vi "DevicePXIStar.vi"(11 "Channel Name":string) -> (2 "Trigger Source":string, 3 "PXIStarLine":string)   [LabVIEW 2014]
doc: "Takes a DAQmx Channel Name identifies the DAQmx device and outputs the device's PXI_Star port line and the PXI_Star line the device is connected to in the chasis.\n\nPXI_Star line of the device is the /\"device_name\"/PXI_Star \nPXI_Star line number is the slot number of the device minus 3."
uses:
  <resource>/objmgr/daqmx.rc
panel:
  out "PXI/PCI Settings:Slot Path":string
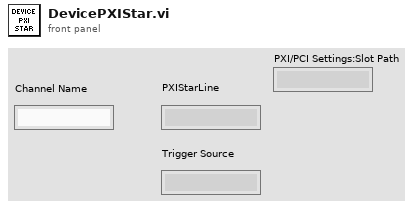
[diagram p1: front panel]
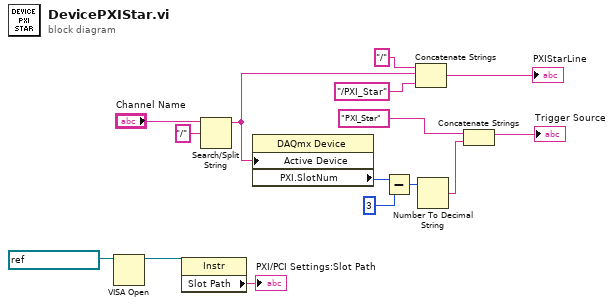
[diagram p0: block diagram]
diagram:
  n1 = VISA Open(VISA resource name=refnum<visa-resource-name> "RIO0::INSTR") -> (VISA resource name=w3:refnum<visa-resource-name>)  [unwired: 4 in, 1 out]
  n2 = property class="Instr"(reference=w3) -> ("Slot Path"=→"PXI/PCI Settings:Slot Path":string)  [unwired: 1 in, 2 out]
  n3 = Search/Split String(string="Channel Name", search string/char (-)="/") -> (substring before match=w6:string)  [unwired: 1 in, 2 out]
  n4 = property class="DAQmx Device"("Active Device"=w6) -> ("PXI.SlotNum"=w10:u32)  [unwired: 2 in, 2 out]
  n5 = Subtract(x=w10, y=u32 3) -> (x-y=w12:u32)
  n6 = Concatenate Strings("/" ("string"), w6, "/PXI_Star" ("string")) -> (→"PXIStarLine":string)
  n7 = Number To Decimal String(number=w12) -> (decimal integer string=w13:string)  [unwired: 1 in]
  n8 = Concatenate Strings("PXI_Star" ("string"), w13) -> (→"Trigger Source":string)
